vi "Read.vi"(8 "error in (no error)":errorcluster caption="entrée d'erreur (pas d'erreur)", 11 "Class UART Nodon.lvclass En entrée":refnum<class "Class UART Zigbee.lvclass">) -> (0 "error out":errorcluster caption="sortie d'erreur", 3 "Class UART Nodon.lvclass En sortie":refnum<class "Class UART Zigbee.lvclass">)   [LabVIEW 2020, in "Library Instrument & Equipement.lvlib" / "Library UART.lvlib" / "Class UART Zigbee.lvclass"]
uses:
  Class UART Zigbee.lvclass
  C:/Users/ngarcin/OneDrive - Altyor/Standard TB/Class/UART/UART (Default)/Class UART (Default).lvclass
  Class UART Zigbee.lvclass/Class UART Zigbee.ctl
  Commun VI/Library Commun.lvlib
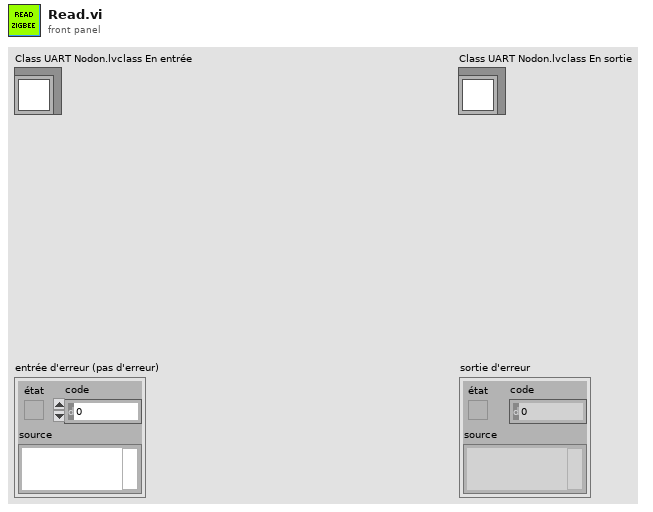
[diagram p1: front panel]
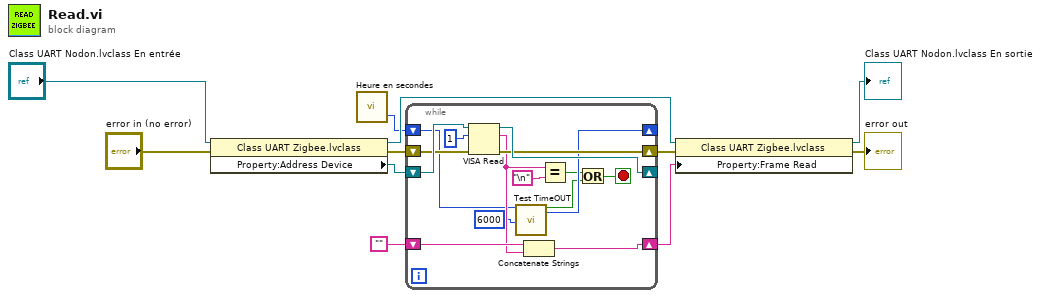
[diagram p0: block diagram]
diagram:
  n1 = property class="Class UART Zigbee.lvclass"(reference="Class UART Nodon.lvclass En entrée", error in="error in (no error)") -> (reference out=w5:refnum<class "Class UART Zigbee.lvclass">, error out=w8:errorcluster, "Property:Address Device"=w9:refnum<visa-resource-name>)
  n2 = call "Heure en secondes.vi"() -> ("Heure en milisecondes"=w1:u32)  [unwired: 2 in, 1 out]
  n3 = while {
    shift-right: [w22] -> _
    shift-left: w9 -> [w25]
    shift-right: [w21] -> w2
    shift-left: w8 -> [w24]
    shift-right: [w18] -> w3
    shift-left: "" -> [w20]
    shift-right: [w16] -> _
    shift-left: w1 -> [w17]
    stop <- w13 stop-if-true
    n4 = VISA Read(VISA resource name=w25, byte count=u32 1 ("nombre d'octets"), error in (no error)=w24) -> (VISA resource name out=w22:refnum<visa-resource-name>, read buffer=w19:string, error out=w21:errorcluster)  [unwired: 1 out]
    n5 = call "Test TimeOUT.vi"("OLD Time"=w17, "TimeOut ms"=u32 6000) -> ("Timeout ?"=w12:bool, "NEW Time"=w16:u32)  [unwired: 13 in, 3 out]
    n6 = Concatenate Strings(w20, w19) -> (w18:string)
    n7 = Equal?(x=w19, y="\n") -> (x = y?=w14:bool)
    n8 = Or(x=w14, y=w12) -> (x .or. y?=w13:bool)
  }
  n9 = property class="Class UART Zigbee.lvclass"(reference=w5, error in=w2, "Property:Frame Read"=w3) -> (reference out=→"Class UART Nodon.lvclass En sortie":refnum<class "Class UART Zigbee.lvclass">, error out=→"error out":errorcluster)
